vi "getSubordinates.vi"(8 "error in (no error)":errorcluster, 11 "Composite Employee in":refnum<class "Composite Employee.lvclass">) -> (0 "error out":errorcluster, 2 "subordinates":refnum<class "Employee.lvclass">[](array[class]), 3 "Composite Employee out":refnum<class "Composite Employee.lvclass">)   [LabVIEW 2016, in "Composite Employee.lvclass"]
uses:
  Composite Employee.lvclass
  Employee Class/Employee.lvclass
  Composite Employee.lvclass/Composite Employee.ctl
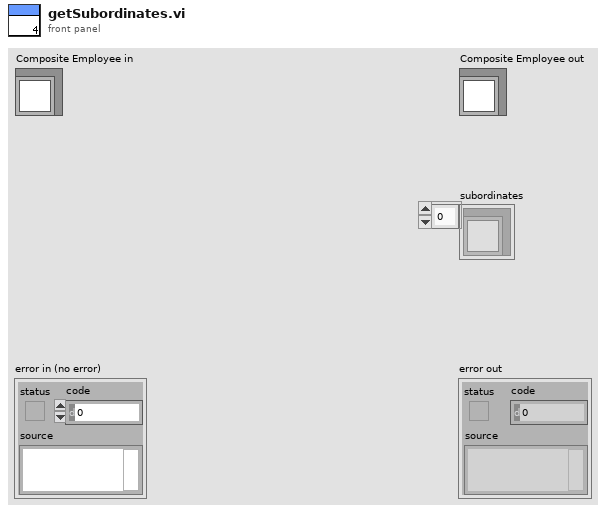
[diagram p1: front panel]
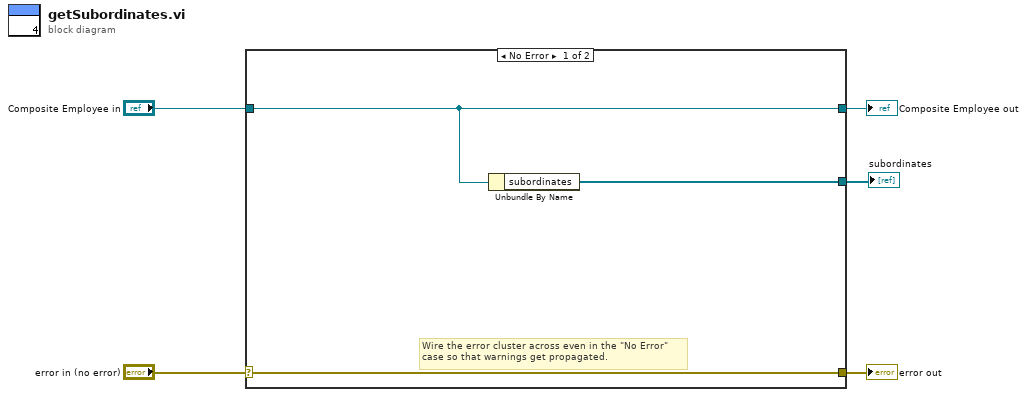
[diagram p0: block diagram]
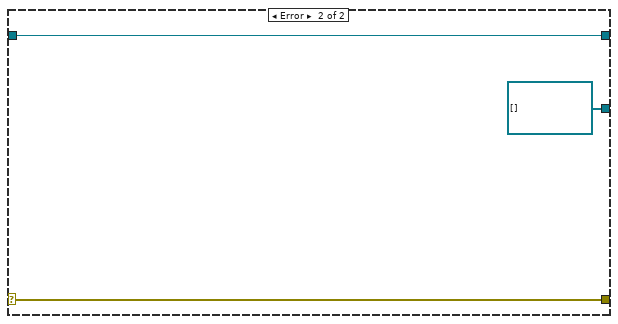
[diagram p2: hidden frame]
diagram:
  n1 = case shown="No Error" "error in (no error)" {
    selector: "error in (no error)" -> [w8 w11]
    tunnel: [w8 w11] -> w4
    tunnel: [w7 w10] -> w2
    tunnel: "Composite Employee in" -> [w7 w10]
    tunnel: [w6 refnum<class "Employee.lvclass">[] [] ("subordinates")] -> w1
    frame No Error {
      # "Wire the error cluster across even in the \"No Error\"\ncase so that warnings get propagated."
      n2 = Unbundle By Name(w7) -> ("subordinates"=w6:refnum<class "Employee.lvclass">[])
    }
    frame Error {
    }
  }
  "error out" <- w4
  "Composite Employee out" <- w2
  "subordinates" <- w1
